vi "FrameGraber.vi"(0 "Exposure Time":dbl=16602.0 min=56.0 max=16602.0, 1 "Gain":dbl=2.6607250597988097 min=1.0 max=3.9810717055349722, 5 "Stop (F)":bool, 7 "error in":errorcluster) -> (20 "Image Out":T1(plugin-control), 22 "Image Number":u32, 25 "Frame Rate":dbl, 26 "Stopped":bool, 27 "error out":errorcluster)   [LabVIEW 2011]
doc: "Creates, and edits acquisitions using the NI Vision Acquisition Express VI.\n\nThe NI Vision Acquisition Wizard is launched by placing the Express VI on the block diagram. Select an acquisition source and configure an acquisition using NI-IMAQ, NI-IMAQdx, or simulate an acquisition by reading an AVI or image files from a folder. After an acquisition is configured, select controls and indicators to be able to programmatically set in LabVIEW. Double-click the Vision Acquisition Express VI to edit the acquisition.\n\nNote: Any images created by the Express VI need to be disposed after use. Use the IMAQ Dispose.vi to cleanup the images output by the Express VI when they are no longer needed."
uses:
  <vilib>/vision/driver/NI_Vision_Acquisition_Software.lvlib
  C:/Program Files/National Instruments/LabVIEW 2011/resource/objmgr/imaqdx.rc
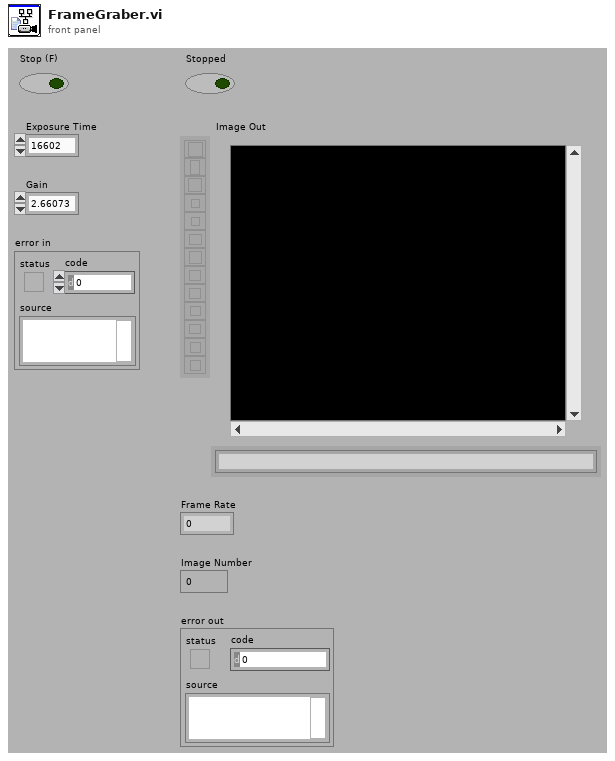
[diagram p1: front panel]
types:
  T1 = typedef "IMAQ Image.ctl" = refnum<image>
  T2 = typedef "IMAQdx.ctl" = refnum<k21>
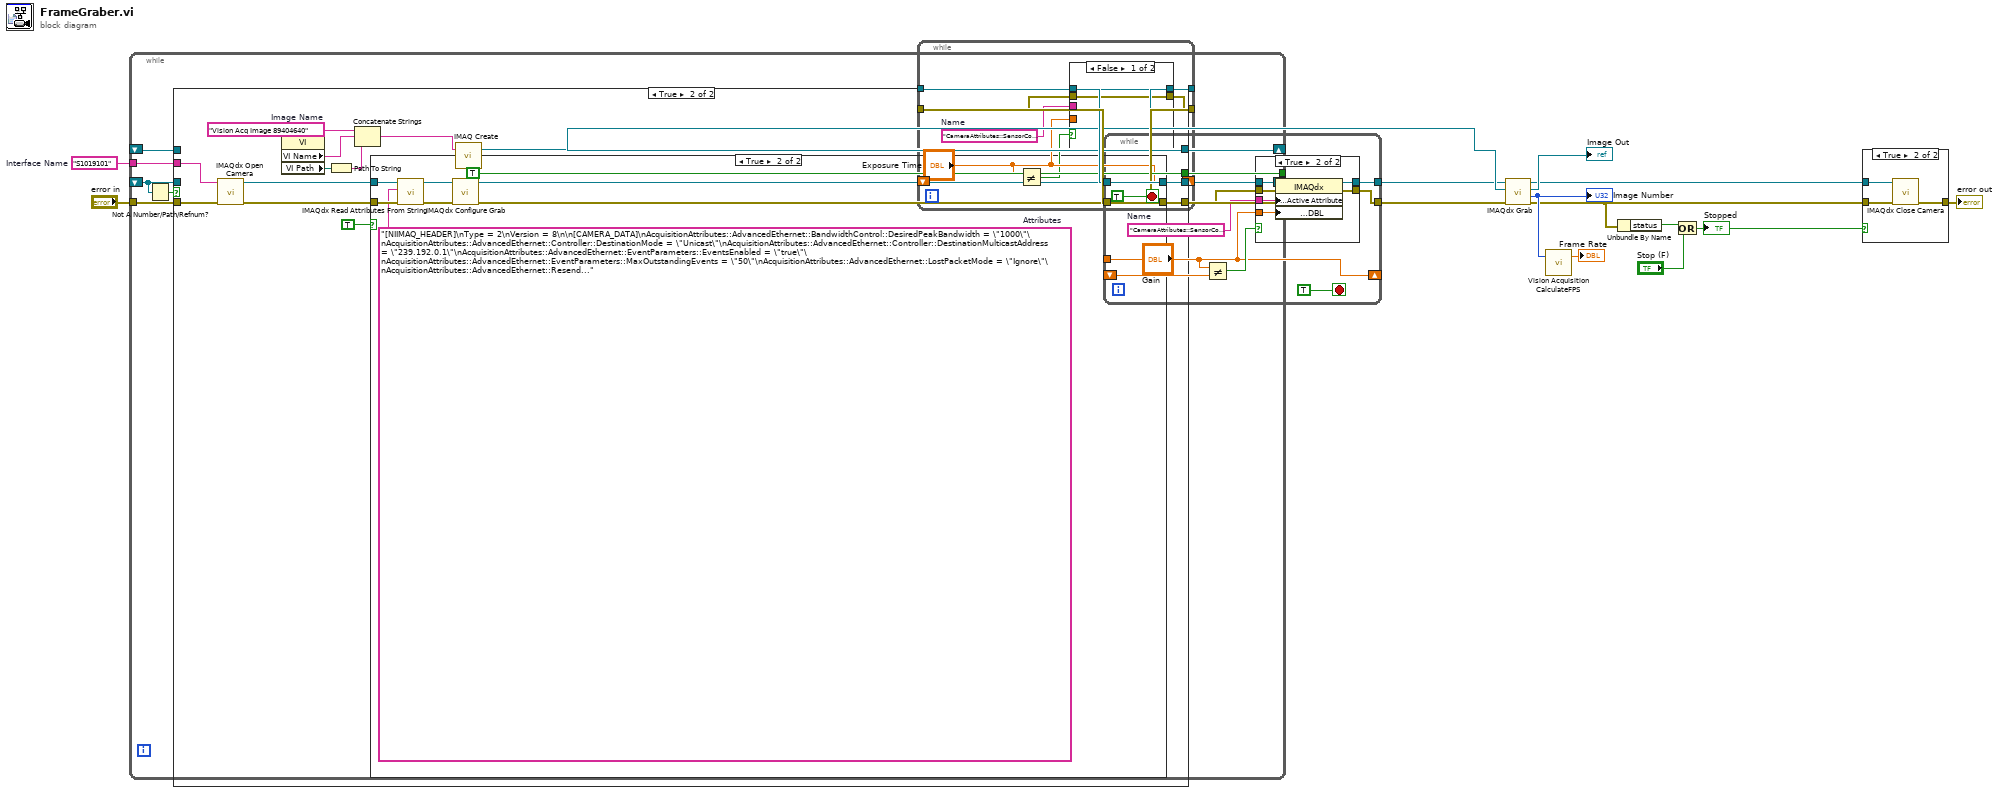
[diagram p0: block diagram]
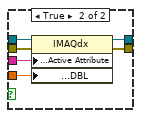
[diagram p4: hidden frame]
diagram:
  w16 = "S1019101"  # Interface Name
  n1 = while "While Loop_template0" {
    shift-right: [w28] -> w15
    shift-left: _ -> [w21]
    tunnel: [w27] -> w17
    tunnel: "error in" -> [w26]
    shift-right: [w24] -> w6
    shift-left: _ -> [w23]
    tunnel: w16 -> [w22]
    tunnel: [w19] -> _
    stop <- TRUE ("_template0") stop-if-true
    n2 = Not A Number/Path/Refnum?(number/path/refnum=w21) -> (NaN/Path/Refnum?=w20:bool)
    n3 = case "Case Structure_template0" shown="True" w20 {
      tunnel: [w31 w46] -> w28
      tunnel: w21 -> [w31 _]
      tunnel: [w30 w45] -> w27
      tunnel: w26 -> [w30 w47]
      tunnel: [w29 w44] -> w24
      tunnel: w23 -> [w29 _]
      tunnel: w22 -> [_ w34]
      tunnel: [_ TRUE] -> w19
      frame False {
      }
      frame True {
        w39 = "Vision Acq Image 89404640"  # Image Name
        n4 = call <vilib>:"IMAQdx Open Camera.vi"("error in"=w47, "Session In"=w34) -> ("error out"=w37:errorcluster, "Session Out"=w38:T2)  [unwired: 1 in, 7 out]
        n5 = property class="VI"() -> ("VI Name"=w42:string, "VI Path"=w43:path)  [unwired: 2 in, 2 out]
        n6 = Path To String(path=w43) -> (string=w41:string)
        n7 = Concatenate Strings(w39, w42, w41) -> (w40:string)
        n8 = case shown="True" TRUE ("Init Attributes") {
          tunnel: w38 -> [w49 w54]
          tunnel: w37 -> [w48 w53]
          tunnel: [w49 w51] -> w36
          tunnel: [w48 w50] -> w35
          frame False {
          }
          frame True {
            w52 = "[NIIMAQ_HEADER]\nType = 2\nVersion = 8\n\n[CAMERA_DATA]\nAcquisitionAttributes::AdvancedEthernet::BandwidthControl::DesiredPeakBandwidth = \"1000\"\nAcquisitionAttributes::AdvancedEthernet::Controller::DestinationMode = \"Unicast\"\nAcquisitionAttributes::AdvancedEthernet::Controller::DestinationMulticastAddress = \"239.192.0.1\"\nAcquisitionAttributes::AdvancedEthernet::EventParameters::EventsEnabled = \"true\"\nAcquisitionAttributes::AdvancedEthernet::EventParameters::MaxOutstandingEvents = \"50\"\nAcquisitionAttributes::AdvancedEthernet::LostPacketMode = \"Ignore\"\nAcquisitionAttributes::AdvancedEthernet::ResendParameters::MaxResendsPerPacket = \"25\"\nAcquisitionAttributes::AdvancedEthernet::ResendParameters::MemoryWindowSize = \"1024\"\nAcquisitionAttributes::AdvancedEthernet::ResendParameters::MissingPacketTimeout = \"2\"\nAcquisitionAttributes::AdvancedEthernet::ResendParameters::NewPacketTimeout = \"100\"\nAcquisitionAttributes::AdvancedEthernet::ResendParameters::ResendBatchingPercentage = \"10\"\nAcquisitionAttributes::AdvancedEthernet::ResendParameters::ResendResponseTimeout = \"2\"\nAcquisitionAttributes::AdvancedEthernet::ResendParameters::ResendsEnabled = \"true\"\nAcquisitionAttributes::AdvancedEthernet::ResendParameters::ResendThresholdPercentage = \"5\"\nAcquisitionAttributes::AdvancedEthernet::ResendParameters::ResendTimerResolution = \"1\"\nAcquisitionAttributes::AdvancedEthernet::TestPacketParameters::MaxTestPacketRetries = \"1\"\nAcquisitionAttributes::AdvancedEthernet::TestPacketParameters::TestPacketEnabled = \"true\"\nAcquisitionAttributes::AdvancedEthernet::TestPacketParameters::TestPacketTimeout = \"250\"\nAcquisitionAttributes::AdvancedGenicam::CommandTimeout = \"100\"\nAcquisitionAttributes::Bayer::GainB = \"1\"\nAcquisitionAttributes::Bayer::GainG = \"1\"\nAcquisitionAttributes::Bayer::GainR = \"1\"\nAcquisitionAttributes::Bayer::Pattern = \"Use hardware value\"\nAcquisitionAttributes::BitsPerPixel = \"Use hardware value\"\nAcquisitionAttributes::ChunkDataDecoding::ChunkDataDecodingEnabled = \"false\"\nAcquisitionAttributes::ChunkDataDecoding::MaximumChunkCopySize = \"64\"\nAcquisitionAttributes::IgnoreFirstFrame = \"false\"\nAcquisitionAttributes::OverwriteMode = \"Get Newest\"\nAcquisitionAttributes::PacketSize = \"1000\"\nAcquisitionAttributes::PixelSignedness = \"Signed\"\nAcquisitionAttributes::ReceiveTimestampMode = \"None\"\nAcquisitionAttributes::ShiftPixelBits = \"false\"\nAcquisitionAttributes::SwapPixelBytes = \"false\"\nAcquisitionAttributes::Timeout = \"5000\"\nCameraAttributes::Persistence::CounterResetLineReg = \"0\"\nCameraAttributes::Persistence::CounterResetModeReg = \"0\"\nCameraAttributes::Persistence::PersistenceAcqFrameCount = \"1\"\nCameraAttributes::Persistence::PersistenceAoiHeightReg = \"480\"\nCameraAttributes::Persistence::PersistenceAoiLeftReg = \"0\"\nCameraAttributes::Persistence::PersistenceAoiTopReg = \"0\"\nCameraAttributes::Persistence::PersistenceAoiWidthReg = \"640\"\nCameraAttributes::Persistence::PersistenceBlackLevelReg = \"0\"\nCameraAttributes::Persistence::PersistenceEventSelector = \"FrameTrigger\"\nCameraAttributes::Persistence::PersistenceEventNotificationReg = \"0\"\nCameraAttributes::Persistence::PersistenceEventSelector = \"ExposureStart\"\nCameraAttributes::Persistence::PersistenceEventNotificationReg = \"0\"\nCameraAttributes::Persistence::PersistenceEventSelector = \"ExposureEnd\"\nCameraAttributes::Persistence::PersistenceEventNotificationReg = \"0\"\nCameraAttributes::Persistence::PersistenceEventSelector = \"InvalidFrameTrigger\"\nCameraAttributes::Persistence::PersistenceEventNotificationReg = \"0\"\nCameraAttributes::Persistence::PersistenceEventSelector = \"AcquisitionEnd\"\nCameraAttributes::Persistence::PersistenceEventNotificationReg = \"0\"\nCameraAttributes::Persistence::PersistenceEventSelector = \"FrameTrigger\"\nCameraAttributes::Persistence::PersistenceExposureAlignmentReg = \"0\"\nCameraAttributes::Persistence::PersistenceFrameRateReg = \"59670\"\nCameraAttributes::Persistence::PersistenceGainReg = \"85\"\nCameraAttributes::Persistence::PersistenceGevConterSource = \"0000000000000000\"\nCameraAttributes::Persistence::PersistenceHorizontalBinningReg = \"1\"\nCameraAttributes::Persistence::PersistenceInput_first = \"0000000000000000\"\nCameraAttributes::Persistence::PersistenceInput_second = \"0100000001000000\"\nCameraAttributes::Persistence::PersistenceLuminanceLut = \"00000100020003000400050006000700080009000A000B000C000D000E000F0010001100120013001400150016001700180019001A001B001C001D001E001F0020002100220023002400250026002700280029002A002B002C002D002E002F0030003100320033003400350036003700380039003A003B003C003D003E003F0040004100420043004400450046004700480049004A004B004C004D004E004F0050005100520053005400550056005700580059005A005B005C005D005E005F0060006100620063006400650066006700680069006A006B006C006D006E006F0070007100720073007400750076007700780079007A007B007C007D007E007F0080008100820083008400850086008700880089008A008B008C008D008E008F0090009100920093009400950096009700980099009A009B009C009D009E009F00A000A100A200A300A400A500A600A700A800A900AA00AB00AC00AD00AE00AF00B000B100B200B300B400B500B600B700B800B900BA00BB00BC00BD00BE00BF00C000C100C200C300C400C500C600C700C800C900CA00CB00CC00CD00CE00CF00D000D100D200D300D400D500D600D700D800D900DA00DB00DC00DD00DE00DF00E000E100E200E300E400E500E600E700E800E900EA00EB00EC00ED00EE00EF00F000F100F200F300F400F500F600F700F800F900FA00FB00FC00FD00FE00FF0000010101020103010401050106010701080109010A010B010C010D010E010F0110011101120113011401150116011701180119011A011B011C011D011E011F0120012101220123012401250126012701280129012A012B012C012D012E012F0130013101320133013401350136013701380139013A013B013C013D013E013F0140014101420143014401450146014701480149014A014B014C014D014E014F0150015101520153015401550156015701580159015A015B015C015D015E015F0160016101620163016401650166016701680169016A016B016C016D016E016F0170017101720173017401750176017701780179017A017B017C017D017E017F0180018101820183018401850186018701880189018A018B018C018D018E018F0190019101920193019401950196019701980199019A019B019C019D019E019F01A001A101A201A301A401A501A601A701A801A901AA01AB01AC01AD01AE01AF01B001B101B201B301B401B501B601B701B801B901BA01BB01BC01BD01BE01BF01C001C101C201C301C401C501C601C701C801C901CA01CB01CC01CD01CE01CF01D001D101D201D301D401D501D601D701D801D901DA01DB01DC01DD01DE01DF01E001E101E201E301E401E501E601E701E801E901EA01EB01EC01ED01EE01EF01F001F101F201F301F401F501F601F701F801F901FA01FB01FC01FD01FE01FF0100020102020203020402050206020702080209020A020B020C020D020E020F0210021102120213021402150216021702180219021A021B021C021D021E021F0220022102220223022402250226022702280229022A022B022C022D022E022F0230023102320233023402350236023702380239023A023B023C023D023E023F0240024102420243024402450246024702480249024A024B024C024D024E024F0250025102520253025402550256025702580259025A025B025C025D025E025F0260026102620263026402650266026702680269026A026B026C026D026E026F0270027102720273027402750276027702780279027A027B027C027D027E027F0280028102820283028402850286028702880289028A028B028C028D028E028F0290029102920293029402950296029702980299029A029B029C029D029E029F02A002A102A202A302A402A502A602A702A802A902AA02AB02AC02AD02AE02AF02B002B102B202B302B402B502B602B702B802B902BA02BB02BC02BD02BE02BF02C002C102C202C302C402C502C602C702C802C902CA02CB02CC02CD02CE02CF02D002D102D202D302D402D502D602D702D802D902DA02DB02DC02DD02DE02DF02E002E102E202E302E402E502E602E702E802E902EA02EB02EC02ED02EE02EF02F002F102F202F302F402F502F602F702F802F902FA02FB02FC02FD02FE02FF0200030103020303030403050306030703080309030A030B030C030D030E030F0310031103120313031403150316031703180319031A031B031C031D031E031F0320032103220323032403250326032703280329032A032B032C032D032E032F0330033103320333033403350336033703380339033A033B033C033D033E033F0340034103420343034403450346034703480349034A034B034C034D034E034F0350035103520353035403550356035703580359035A035B035C035D035E035F0360036103620363036403650366036703680369036A036B036C036D036E036F0370037103720373037403750376037703780379037A037B037C037D037E037F0380038103820383038403850386038703880389038A038B038C038D038E038F0390039103920393039403950396039703980399039A039B039C039D039E039F03A003A103A203A303A403A503A603A703A803A903AA03AB03AC03AD03AE03AF03B003B103B203B303B403B503B603B703B803B903BA03BB03BC03BD03BE03BF03C003C103C203C303C403C503C603C703C803C903CA03CB03CC03CD03CE03CF03D003D103D203D303D403D503D603D703D803D903DA03DB03DC03DD03DE03DF03E003E103E203E303E403E503E603E703E803E903EA03EB03EC03ED03EE03EF03F003F103F203F303F403F503F603F703F803F903FA03FB03FC03FD03FE03FF03\"\nCameraAttributes::Persistence::PersistenceLutEnableReg = \"0\"\nCameraAttributes::Persistence::PersistenceOutput = \"000000000000000006000000000000000000000064000000000000000100000007000000000000000000000064000000\"\nCameraAttributes::Persistence::PersistencePixelFormatReg = \"17301505\"\nCameraAttributes::Persistence::PersistenceShutterModeReg = \"1\"\nCameraAttributes::Persistence::PersistenceShutterReg = \"6020\"\nCameraAttributes::Persistence::PersistenceTestImageSelectorReg = \"0\"\nCameraAttributes::Persistence::PersistenceTriggerDelayReg = \"100\"\nCameraAttributes::Persistence::PersistenceTriggerModeReg = \"0\"\nCameraAttributes::Persistence::PersistenceTriggerSourceReg = \"0\"\nCameraAttributes::Persistence::PersistenceVerticalBinningReg = \"1\"\n"  # Attributes
            n9 = call <vilib>:"IMAQdx Read Attributes From String.vi"("error in"=w53, "Attributes String In"=w52, "Session In"=w54) -> ("error out"=w50:errorcluster, "Session Out"=w51:T2)  [unwired: 7 out]
          }
        }
        n10 = call <vilib>:"IMAQdx Configure Grab.vi"("error in"=w35, "Session In"=w36) -> ("error out"=w45:errorcluster, "Session Out"=w46:T2)  [unwired: 8 out]
        n11 = call "IMAQ Create"("Image Name"=w40) -> ("New Image"=w44:T1)  [unwired: 3 in, 2 out]
      }
    }
  }
  n12 = while {
    tunnel: w17 -> [w63]
    tunnel: [w62] -> w13
    tunnel: w15 -> [w61]
    tunnel: [w60] -> w14
    shift-right: ["Exposure Time"] -> _
    shift-left: _ -> [w56]
    stop <- TRUE stop-if-true
    w59 = "CameraAttributes::SensorControl::ExposureTimeAbs"  # Name
    n13 = Not Equal?(x="Exposure Time", y=w56) -> (x != y?=w55:bool)
    n14 = case shown="False" w55 {
      tunnel: w63 -> [w64 w71]
      tunnel: [w65 w70] -> w62
      tunnel: w61 -> [w65 w69]
      tunnel: [w64 w68] -> w60
      tunnel: w59 -> [_ w67]
      tunnel: "Exposure Time" -> [_ w66]
      frame False {
      }
      frame True {
        n15 = property class="IMAQdx"(reference=w69, error in=w71, "Camera Attributes:Active Attribute"=w67, "Camera Attributes:Value:DBL"=w66) -> (reference out=w70:T2, error out=w68:errorcluster)
      }
    }
  }
  n16 = while {
    tunnel: w14 -> [w80]
    tunnel: [w79] -> w5
    tunnel: w13 -> [w78]
    tunnel: [w77] -> w12
    shift-right: ["Gain"] -> _
    shift-left: _ -> [w74]
    tunnel: ["Gain"] -> _
    stop <- TRUE stop-if-true
    w76 = "CameraAttributes::SensorControl::GainAbs"  # Name
    n17 = Not Equal?(x="Gain", y=w74) -> (x != y?=w73:bool)
    n18 = case shown="True" w73 {
      tunnel: w80 -> [w81 w88]
      tunnel: [w82 w87] -> w79
      tunnel: w78 -> [w82 w86]
      tunnel: [w81 w85] -> w77
      tunnel: w76 -> [_ w84]
      tunnel: "Gain" -> [_ w83]
      frame False {
      }
      frame True {
        n19 = property class="IMAQdx"(reference=w86, error in=w88, "Camera Attributes:Active Attribute"=w84, "Camera Attributes:Value:DBL"=w83) -> (reference out=w87:T2, error out=w85:errorcluster)
      }
    }
  }
  n20 = call <vilib>:"IMAQdx Grab.vi"("error in"=w12, "Image In"=w6, "Session In"=w5) -> ("error out"=w4:errorcluster, "Buffer Number Out"=w8:u32, "Image Out"=→"Image Out":T1, "Session Out"=w3:T2)  [unwired: 1 in, 4 out]
  "Image Number" <- w8
  n21 = call <vilib>:"Vision Acquisition CalculateFPS.vi"("buffer number"=w8) -> ("acquired FPS"=→"Frame Rate":dbl)  [unwired: 2 out]
  n22 = Unbundle By Name(w4) -> ("status"=w11:bool)
  n23 = Or(x=w11, y="Stop (F)") -> (x .or. y?=w2:bool)
  "Stopped" <- w2
  n24 = case "Case Structure_template1" shown="True" w2 {
    tunnel: [w89 w91] -> w1
    tunnel: w4 -> [w89 w92]
    tunnel: w3 -> [_ w90]
    frame False {
    }
    frame True {
      n25 = call <vilib>:"IMAQdx Close Camera.vi"("error in"=w92, "Session In"=w90) -> ("error out"=w91:errorcluster)  [unwired: 9 out]
    }
  }
  "error out" <- w1
